vi "FTW-Example-Endpoints.vi"() -> ()   [LabVIEW 2013]
uses:
  src/core/actor/endpoint/FTW-Endpoint-MessageTransportScheme.ctl
  src/core/actor/endpoint/FTW-Endpoint-Type.ctl
  src/core/actor/endpoint/FTW-Actor-Endpoint.lvclass
panel:
  out "error out 2":errorcluster
  in  "stop":bool
  out "x+1":i32
  out "millisecond timer value":u32
  out "Response Received?":bool
  out "Request Received?":bool
  in  "Enpoint Type":T1
  out "Endpoint Address":string
  out "error out":errorcluster
  out "Response":string
  out "Request":string
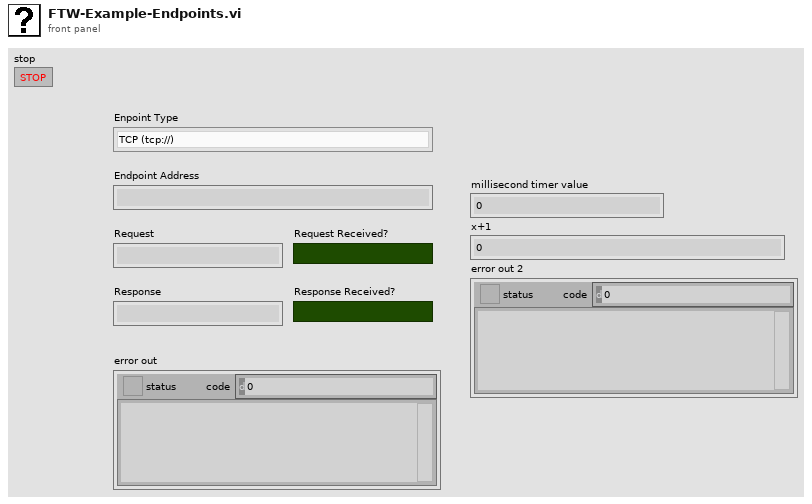
[diagram p1: front panel]
types:
  T1 = typedef "FTW-Actor-Endpoint.lvclass/FTW-Endpoint-MessageTransportScheme.ctl" = enum16{"TCP (tcp://)", "Inter-Process (ipc://)", "In-Process (inproc://)"}
  T2 = typedef "FTW-Actor-Endpoint.lvclass/FTW-Endpoint-Type.ctl" = enum32{"Server", "Client", "Publisher", "Subscriber", "Pipeline Producer", "Pipeline Consumer", "Surveyor", "Respondent", "Exclusive Pair", "Bus"}
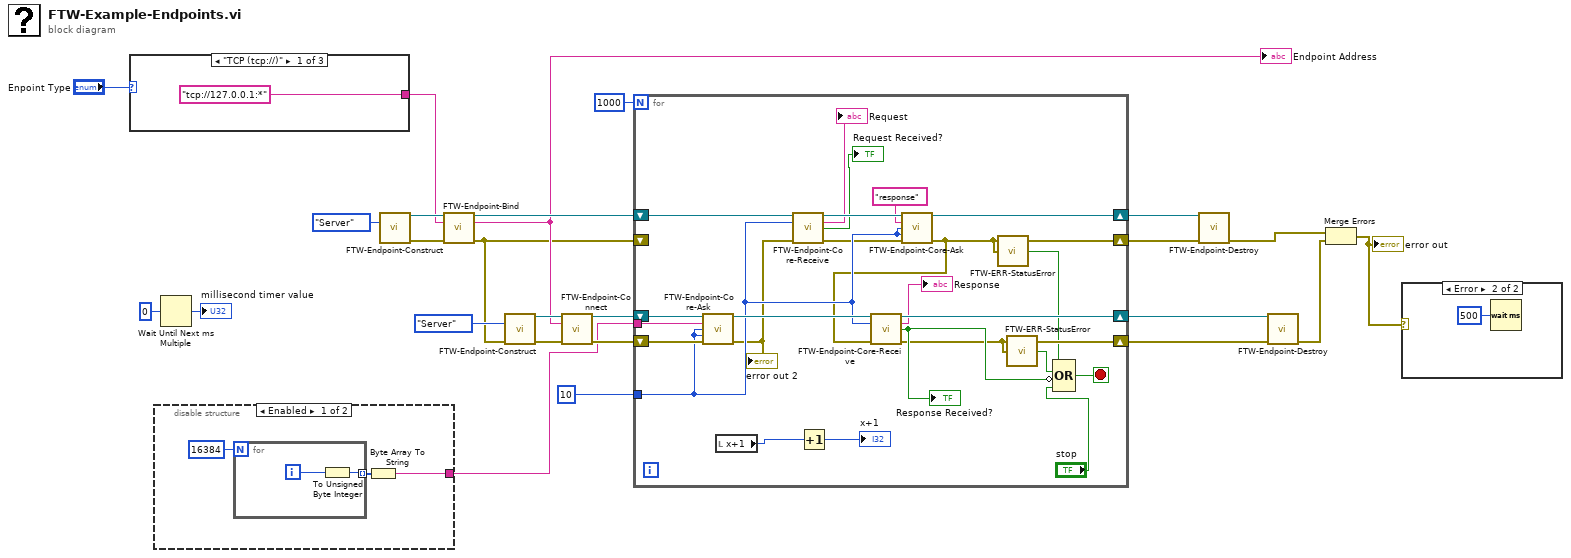
[diagram p0: block diagram]
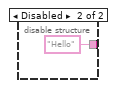
[diagram p2: hidden frame]
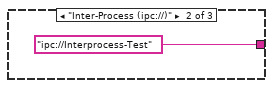
[diagram p4: hidden frame]
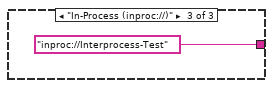
[diagram p5: hidden frame]
diagram:
  n1 = case shown="\"TCP (tcp://)\"" "Enpoint Type" {
    tunnel: ["tcp://127.0.0.1:*" ("Server Address") "ipc://Interprocess-Test" ("Server Address") "inproc://Interprocess-Test" ("Server Address")] -> w20
    frame "TCP (tcp://)" {
    }
    frame "Inter-Process (ipc://)" {
    }
    frame "In-Process (inproc://)" {
    }
  }
  n2 = disable-structure shown="Enabled" {
    disable-tunnel: [w29 "Hello" ("string")] -> w7
    frame Enabled {
      n3 = for {
        N: 16384 -> [_]
        tunnel: [w32] -> w30 mode=indexing
        i -> [w33]
        n4 = To Unsigned Byte Integer(number=w33) -> (unsigned 8bit integer=w32:u8)
      }
      n5 = Byte Array To String(unsigned byte array=w30) -> (string=w29:string)
    }
    frame Disabled {
    }
  }
  n6 = Wait Until Next ms Multiple(millisecond multiple=u32 0 ("milliseconds to wait")) -> (millisecond timer value=→"millisecond timer value":u32)
  n7 = call "FTW-Endpoint-Construct.vi"("Endpoint Type"=FTW-Endpoint-Type."Server") -> ("FTW Endpoint"=w23:refnum<class "FTW-Actor-Endpoint.lvclass">, "error out"=w21:errorcluster)  [unwired: 13 in]
  n8 = call-dynamic "FTW-Endpoint-Bind.vi"("FTW Endpoint"=w23, "Remote Endpoint Address"=w20, "error in"=w21) -> ("FTW Endpoint out"=w22:refnum<class "FTW-Actor-Endpoint.lvclass">, "Actual Endpoint Address"=w15:string, "error out"=w5:errorcluster)  [unwired: 10 in]
  "Endpoint Address" <- w15
  n9 = call "FTW-Endpoint-Construct.vi"("Endpoint Type"=FTW-Endpoint-Type."Server", "error in"=w5) -> ("FTW Endpoint"=w18:refnum<class "FTW-Actor-Endpoint.lvclass">, "error out"=w16:errorcluster)  [unwired: 12 in]
  n10 = call "FTW-Endpoint-Connect.vi"("FTW Socket"=w18, "Remote Address"=w15, "error in"=w16) -> ("FTW Socket out"=w17:refnum<class "FTW-Actor-Endpoint.lvclass">, "error out"=w8:errorcluster)  [unwired: 11 in]
  n11 = for {
    N: 1000 -> [_]
    tunnel: w7 -> [w47]
    tunnel: 10 ("Read Timeout") -> [w46]
    shift-right: [w55] -> w14
    shift-left: w22 -> [w58]
    shift-right: [w53] -> w13
    shift-left: w17 -> [w57]
    shift-right: [w35] -> w4
    shift-left: w5 -> [_]
    shift-right: [w43] -> w3
    shift-left: w8 -> [w48]
    stop <- w40 stop-if-true
    n12 = call "FTW-Endpoint-Core-Ask.vi"("FTW Socket"=w57, "Request"=w47, "Read Timeout"=w46, "Write Timeout"=w46, "error in"=w48) -> ("FTW Socket out"=w54:refnum<class "FTW-Actor-Endpoint.lvclass">, "error out"=w37:errorcluster)  [unwired: 6 in, 3 out]
    "error out 2" <- w37
    n13 = local read "x+1"() -> (w39:i32)
    n14 = call "FTW-Endpoint-Core-Receive.vi"("FTW Endpoint"=w58, "Timeout"=w46, "error in"=w37) -> ("FTW Endpoint out"=w56:refnum<class "FTW-Actor-Endpoint.lvclass">, "Message"=→"Request":string, "Message Received?"=→"Request Received?":bool, "error out"=w36:errorcluster)  [unwired: 7 in, 2 out]
    n15 = Increment(x=w39) -> (x+1=→"x+1":i32)
    n16 = call "FTW-Endpoint-Core-Ask.vi"("FTW Socket"=w56, "Request"="response", "Read Timeout"=w46, "Write Timeout"=w46, "error in"=w36) -> ("FTW Socket out"=w55:refnum<class "FTW-Actor-Endpoint.lvclass">, "error out"=w35:errorcluster)  [unwired: 6 in, 3 out]
    n17 = call "FTW-Endpoint-Core-Receive.vi"("FTW Endpoint"=w54, "Timeout"=w46, "error in"=w35) -> ("FTW Endpoint out"=w53:refnum<class "FTW-Actor-Endpoint.lvclass">, "Message"=→"Response":string, "Message Received?"=w45:bool, "error out"=w43:errorcluster)  [unwired: 7 in, 2 out]
    "Response Received?" <- w45
    n18 = call "FTW-ERR-StatusError.vi"("error to check"=w35) -> ("Error?"=w41:bool)
    n19 = call "FTW-ERR-StatusError.vi"("error to check"=w43) -> ("Error?"=w42:bool)
    n20 = Compound Arithmetic op=OR(w41, w42, invert w45, "stop") -> (w40:bool)
  }
  n21 = call-dynamic "FTW-Endpoint-Destroy.vi"("FTW Socket"=w14, "error in"=w4) -> ("error out"=w2:errorcluster)  [unwired: 13 in]
  n22 = call-dynamic "FTW-Endpoint-Destroy.vi"("FTW Socket"=w13, "error in"=w3) -> ("error out"=w10:errorcluster)  [unwired: 13 in]
  n23 = Merge Errors(w2, w10) -> (w9:errorcluster)
  "error out" <- w9
  n24 = case shown="Error" w9 {
    frame No Error {
    }
    frame Error {
      n25 = Wait (ms)(milliseconds to wait=u32 500) -> ()  [unwired: 1 out]
    }
  }
